vi "Test 2 port TX RX.vi"() -> ()   [LabVIEW 2021]
uses:
  typedef/CAN Port Configuration.ctl
  typedef/CAN Mode.ctl
  typedef/FD Config.ctl
  Channels/ChannelRegistrar/typedef/Datatype CAN.ctl
  CAN_Logic.lvclass/CAN_Logic.ctl
  Decode Tags.vi
  <vilib>/Utility/error.llb/Clear Errors.vi
  CIFUtilities/CIFClocks/Time Conversion/LabVIEW Time to UTC Time.vi
  Encode Tags.vi
  <vilib>/xnet/xnet.llb/XNET Write.vi
  <vilib>/xnet/xnet.llb/XNET Write (Frame CAN).vi
  <vilib>/xnet/xnet.llb/XNET Read.vi
  <vilib>/xnet/xnet.llb/XNET Read (Frame CAN).vi
  CAN_Logic.lvclass
  Channels/ChannelRegistrar/ChannelRegistrar.lvlib
panel:
  out "CAN Data 2":T1[](array[typedef]) {"Tags" format="%.0x"; "payload" format="%x"; "identifier" format="%x"}
  out "error out":errorcluster
  in  "CAN Data":T1[](array[typedef])=[{"payload"=[0, 0, 0, 0, 0, 0, 0, 51], "identifier"=1, "Tags"=0, "Timestamp"=0}, {"payload"=[0, 0, 0, 0, 0, 0, 0, 36], "identifier"=2, "Tags"=0, "Timestamp"=0}] {"Tags" format="%.0x"; "payload" format="%x"; "identifier" format="%x"}
  in  "Port Configuration":T2={"Mode"=enum."CAN FD", "Baud Rate"=500000, "Temination On"=TRUE, "Subordinate"=FALSE, "Echo TX"=FALSE, "FD Config"={"FD Baud Rate"=2000000, "ISO Mode"=TRUE, "BRS Enabled"=TRUE}} {"FD Config"."FD Baud Rate" format="%.0p"; "Baud Rate" format="%.0p"}
  in  "RX Initerface":string="CAN2"
  in  "TX Interface":string="CAN1"
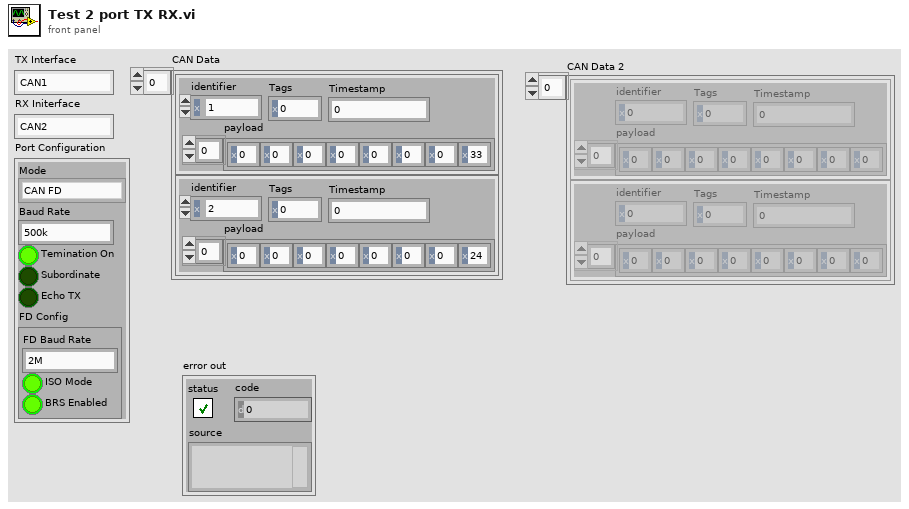
[diagram p1: front panel]
types:
  T1 = typedef "ChannelRegistrar.lvlib/Datatype CAN.ctl" = cluster{"payload":u8[], "identifier":u32, "Tags":u8, "Timestamp":u64}
  T2 = typedef "CAN_Logic.lvclass/CAN Port Configuration.ctl" = cluster{"Mode":T3, "Baud Rate":u64, "Temination On":bool, "Subordinate":bool, "Echo TX":bool, "FD Config":T4}
  T3 = typedef "CAN_Logic.lvclass/CAN Mode.ctl" = enum16{"CAN 2.0", "CAN FD"}
  T4 = typedef "CAN_Logic.lvclass/FD Config.ctl" = cluster{"FD Baud Rate":u64, "ISO Mode":bool, "BRS Enabled":bool}
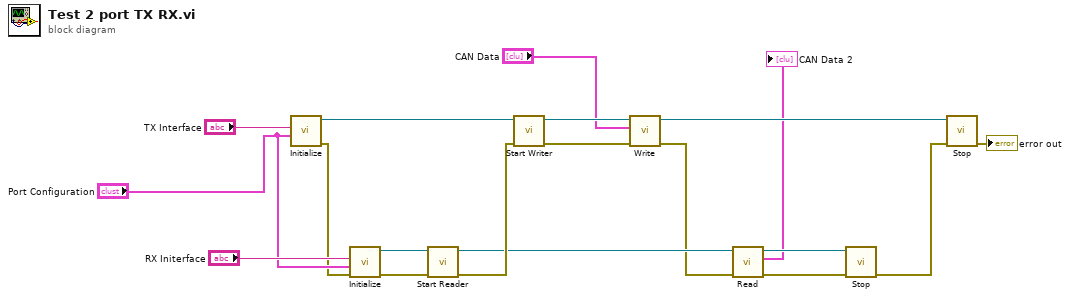
[diagram p0: block diagram]
diagram:
  n1 = call "Initialize.vi"("Port Configuration"="Port Configuration", "Interface"="TX Interface") -> ("error out"=w16:errorcluster, "CAN_Logic out"=w15:refnum<class "CAN_Logic.lvclass">)  [unwired: 8 in]
  n2 = call "Initialize.vi"("error in (no error)"=w16, "Port Configuration"="Port Configuration", "Interface"="RX Initerface") -> ("error out"=w13:errorcluster, "CAN_Logic out"=w14:refnum<class "CAN_Logic.lvclass">)  [unwired: 7 in]
  n3 = call "Start Reader.vi"("error in (no error)"=w13, "CAN_Logic in"=w14) -> ("error out"=w12:errorcluster, "CAN_Logic out"=w8:refnum<class "CAN_Logic.lvclass">)  [unwired: 8 in]
  n4 = call "Start Writer.vi"("error in (no error)"=w12, "CAN_Logic in"=w15) -> ("error out"=w10:errorcluster, "CAN_Logic out"=w11:refnum<class "CAN_Logic.lvclass">)  [unwired: 8 in]
  n5 = call "Write.vi"("error in (no error)"=w10, "CAN Data"="CAN Data", "CAN_Logic in"=w11) -> ("error out"=w7:errorcluster, "CAN_Logic out"=w3:refnum<class "CAN_Logic.lvclass">)  [unwired: 7 in]
  n6 = call "Read.vi"("error in (no error)"=w7, "CAN_Logic in"=w8) -> ("error out"=w5:errorcluster, "CAN Data"=→"CAN Data 2":T1[], "CAN_Logic out"=w6:refnum<class "CAN_Logic.lvclass">)  [unwired: 6 in, 1 out]
  n7 = call "Stop.vi"("error in (no error)"=w5, "CAN_Logic in"=w6) -> ("error out"=w4:errorcluster)  [unwired: 8 in, 1 out]
  n8 = call "Stop.vi"("error in (no error)"=w4, "CAN_Logic in"=w3) -> ("error out"=→"error out":errorcluster)  [unwired: 8 in, 1 out]
